vi "Extract data until pattern.vi"(8 "error in (no error)":errorcluster, 10 "pattern to match":string="\r\n\r\n", 11 "Queue in":refnum<queue>) -> (0 "error out":errorcluster, 2 "Data until pattern (inclusive)":string, 3 "Queue out":refnum<queue>)   [LabVIEW 2013]
uses:
  <vilib>/regexp/Match Regular Expression.xnode
panel:
  out "i":i32
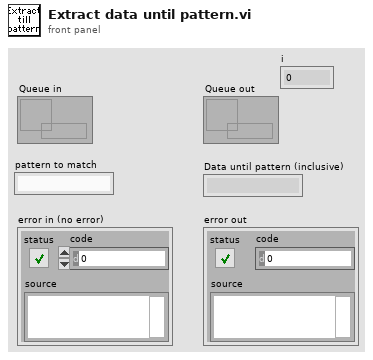
[diagram p1: front panel]
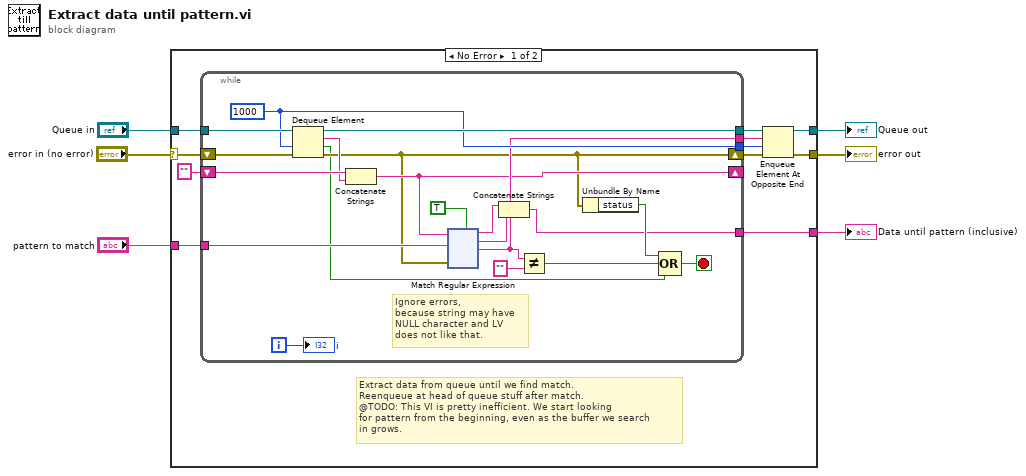
[diagram p0: block diagram]
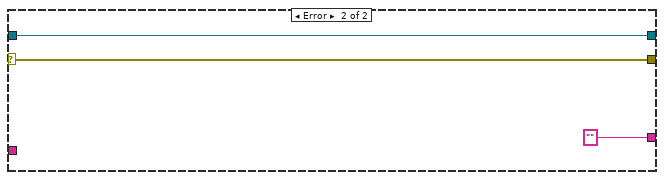
[diagram p2: hidden frame]
diagram:
  n1 = case shown="No Error" "error in (no error)" {
    selector: "error in (no error)" -> [w11 w154]
    tunnel: [w17 w154] -> w6
    tunnel: [w15 w153] -> w5
    tunnel: [w13 "" ("before match")] -> w4
    tunnel: "Queue in" -> [w12 w153]
    tunnel: "pattern to match" -> [w9 _]
    frame No Error {
      # "Extract data from queue until we find match.\nReenqueue at head of queue stuff after match.\n@TODO: This VI is pretty inefficient. We start looking\nfor pattern from the beginning, even as the buffer we search\nin grows."
      n2 = while {
        tunnel: [w31] -> w16
        tunnel: [w37] -> w14
        tunnel: [w21] -> w13
        tunnel: w12 -> [w36]
        tunnel: [w34] -> w10
        tunnel: w9 -> [w33]
        shift-right: [w26] -> _
        shift-left: "" ("y") -> [w28]
        shift-right: [w25] -> w8
        shift-left: w11 -> [w35]
        i -> [w29]
        stop <- w22 stop-if-true
        w34 = 1000 ("timeout in ms (-1)")
        # "Ignore errors,\nbecause string may have\nNULL character and LV \ndoes not like that."
        n3 = Dequeue Element(queue=w36, timeout in ms (-1)=w34, error in (no error)=w35) -> (queue out=w37:refnum<queue>, element=w27:string, timed out?=w18:bool, error out=w25:errorcluster)
        n4 = Concatenate Strings(w28, w27) -> (w26:string)
        n5 = xnode "Match Regular Expression"("input string"=w26, "regular expression"=w33, "error in"=w25, "multiline? (F)"=TRUE) -> ("before match"=w20:string, "whole match"=w19:string, "after match"=w31:string)  [unwired: 2 in, 2 out]
        n6 = Concatenate Strings(w20, w19) -> (w21:string)
        n7 = Not Equal?(x=w31, y="") -> (x != y?=w23:bool)
        n8 = Unbundle By Name(w25) -> ("status"=w24:bool)
        n9 = Compound Arithmetic op=OR(w24, w23, w18) -> (w22:bool)
        "i" <- w29
      }
      n10 = Enqueue Element At Opposite End(queue=w14, element=w16, timeout in ms (-1)=w10, error in (no error)=w8) -> (queue out=w15:refnum<queue>, error out=w17:errorcluster)  [unwired: 1 out]
    }
    frame Error {
    }
  }
  "error out" <- w6
  "Queue out" <- w5
  "Data until pattern (inclusive)" <- w4
